vi "Example of JOBJ Tag.vi"() -> ()   [LabVIEW 2019]
doc: "Example of using an <JOBJ> tag to read a JSON Object in that an Array-of-Clusters format. \n\nThis allows handling of JSON Objects with unknown or variable names in a \nformat that LabVIEW can use."
uses:
  a1a0f041-c5c1-43a1-a76d-f3e390036e8a.vi
  8c9053c6-7367-45ea-a096-853d532a0fb8.vi
  vi.lib/JDP Science/JSONtext/JSON text to Variant.vi
  vi.lib/JDP Science/JSONtext/Variant to JSON Text.vi
  vi.lib/JDP Science/JSONtext/LVClass Serializer/JSONtext LVClass Serializer.lvclass
panel:
  out "<JSON> with item added":string
  out "error out":errorcluster
  out "Data":T1
  in  "Example JSON (unknown item names)":string="{\"Config\":{\r    \"A1\":{\"A\":\"dsgfsdgdsg\",\"B\":0},\r    \"A2\":{\"A\":\"sdfdsfsdfs\",\"B\":22},\r    \"A3\":{\"A\":\"fbdfdfbbc\",\"B\":123}\r    },\n   \"Other Stuff\":1\n}"
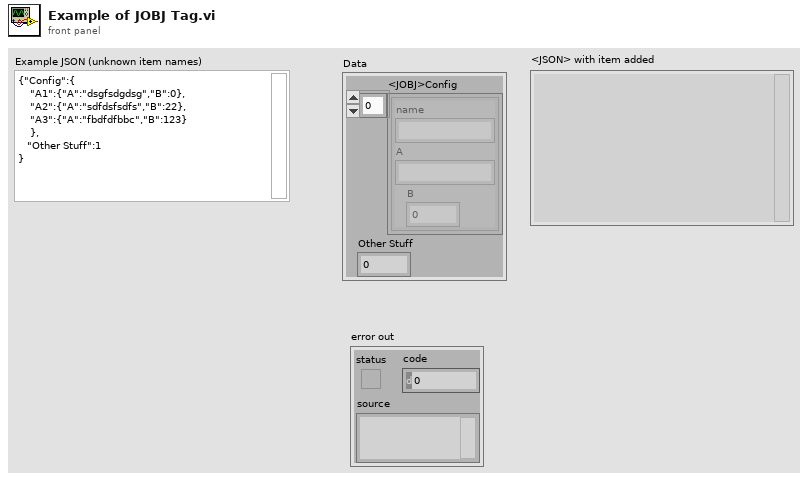
[diagram p1: front panel]
types:
  T1 = cluster{"<JOBJ>Config":cluster{"name":string, "A":string, "B":dbl}[], "Other Stuff":dbl}
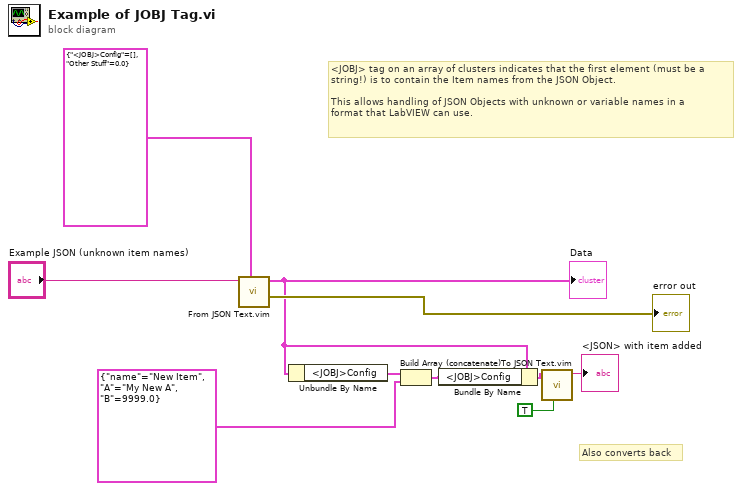
[diagram p0: block diagram]
diagram:
  # "Also converts back"
  # "<JOBJ> tag on an array of clusters indicates that the first element (must be a\nstring!) is to contain the Item names from the JSON Object.\n\nThis allows handling of JSON Objects with unknown or variable names in a \nformat that LabVIEW can use."
  n1 = call "From JSON Text.vim"("Data Type and Default Value"=T1 {"<JOBJ>Config"=[], "Other Stuff"=0.0}, "JSON"="Example JSON (unknown item names)") -> ("error out"=→"error out":errorcluster, "Data out"=w3:T1)  [unwired: 8 in]
  "Data" <- w3
  n2 = Unbundle By Name(w3) -> ("<JOBJ>Config"=w5:cluster{"name":string, "A":string, "B":dbl}[])
  n3 = Build Array (concatenate)(w5, cluster{"name":string, "A":string, "B":dbl} {"name"="New Item", "A"="My New A", "B"=9999.0} ("<JOBJ>Config")) -> (w2:cluster{"name":string, "A":string, "B":dbl}[])
  n4 = Bundle By Name(cluster=w3, "<JOBJ>Config"=w2) -> (w4:T1)
  n5 = call "To JSON Text.vim"("Pretty Print?"=TRUE, "Anything"=w4) -> ("<JSON>"=→"<JSON> with item added":string)  [unwired: 8 in, 1 out]
